vi "IFilterMoveToPosition.vi"(3 "Wheel":i32=2, 4 "filter":i32=2, 5 "PRIORLib.IFilterIn":refnum<k7>) -> (0 "Position":i16, 1 "error out":errorcluster, 2 "PRIORLib.IFilterOut":refnum<k7>)   [LabVIEW 2012]
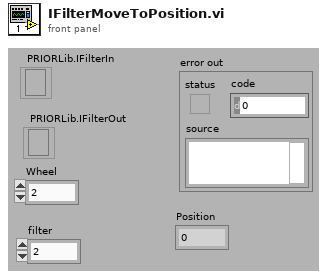
[diagram p1: front panel]
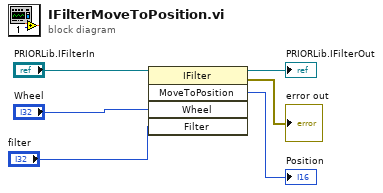
[diagram p0: block diagram]
diagram:
  n1 = invoke class="IFilter" method="MoveToPosition"(reference="PRIORLib.IFilterIn", "Wheel"="Wheel", "Filter"="filter") -> (reference out=→"PRIORLib.IFilterOut":refnum<k7>, error out=→"error out":errorcluster, "MoveToPosition"=→"Position":i32)  [unwired: 2 in, 2 out]
